vi "Systems_WriteConfig.vi"(4 "error in (no error)":errorcluster, 7 "configuration file path":path) -> (0 "error out":errorcluster)   [LabVIEW 2015]
doc: "Write the current engineering settings to the INI file supplied by \"configuration file path\""
uses:
  <vilib>/Utility/config.llb/NI_LVConfig.lvlib
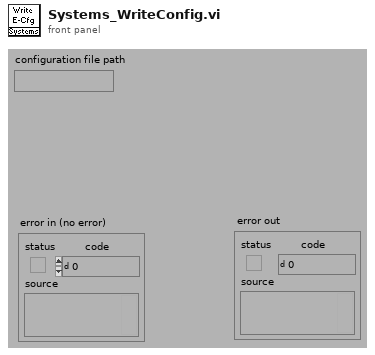
[diagram p1: front panel]
types:
  T1 = typedef "NI_LVConfig.lvlib/Config Data RefNum.ctl" = refnum<k1>
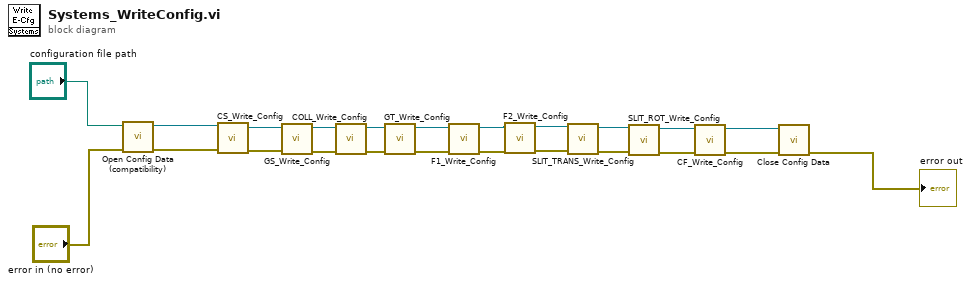
[diagram p0: block diagram]
diagram:
  n1 = call <vilib>:"Open Config Data (compatibility).vi"("error in (no error)"="error in (no error)", "configuration file path"="configuration file path") -> ("error out"=w5:errorcluster, "refnum"=w6:T1)  [unwired: 7 in, 1 out]
  n2 = call "CS_Write_Config.vi"("error in (no error)"=w5, "Config refnum"=w6) -> ("error out"=w8:errorcluster, "refnum out"=w7:T1)  [unwired: 4 in]
  n3 = call "GS_Write_Config.vi"("error in (no error)"=w8, "Config Refnum"=w7) -> ("error out"=w9:errorcluster, "refnum out"=w10:T1)  [unwired: 4 in]
  n4 = call "COLL_Write_Config.vi"("error in (no error)"=w9, "Config Refnum"=w10) -> ("error out"=w11:errorcluster, "refnum out"=w12:T1)  [unwired: 4 in]
  n5 = call "GT_Write_Config.vi"("error in (no error)"=w11, "Config Refnum"=w12) -> ("error out"=w22:errorcluster, "refnum out"=w23:T1)  [unwired: 4 in]
  n6 = call "F1_Write_Config.vi"("error in (no error)"=w22, "Config Refnum"=w23) -> ("error out"=w20:errorcluster, "refnum out"=w21:T1)  [unwired: 4 in]
  n7 = call "F2_Write_Config.vi"("error in (no error)"=w20, "Config Refnum"=w21) -> ("error out"=w18:errorcluster, "refnum out"=w19:T1)  [unwired: 4 in]
  n8 = call "SLIT_TRANS_Write_Config.vi"("error in (no error)"=w18, "Config Refnum"=w19) -> ("error out"=w16:errorcluster, "refnum out"=w17:T1)  [unwired: 4 in]
  n9 = call "SLIT_ROT_Write_Config.vi"("error in (no error)"=w16, "Config Refnum"=w17) -> ("error out"=w3:errorcluster, "refnum out"=w4:T1)  [unwired: 4 in]
  n10 = call "CF_Write_Config.vi"("error in (no error)"=w3, "Config Refnum"=w4) -> ("error out"=w2:errorcluster, "refnum out"=w1:T1)  [unwired: 4 in]
  n11 = call <vilib>:"Close Config Data.vi"("error in (no error)"=w2, "refnum"=w1) -> ("error out"=→"error out":errorcluster)  [unwired: 8 in, 1 out]
